vi "Global 1.vi"() -> ()   [LabVIEW 2015]
panel:
  out "Cam X Pos":dbl
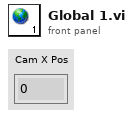
[diagram p1: front panel]
diagram:
